vi "Online_Target_3.vi"   [LabVIEW 2021]
uses:
  Model_Updating_Classes/DROPBEAR_Model_Updating/DROPBEAR_Model_Updating.lvclass
types:
  T1 = cluster{"beam_length":dbl, "youngs_modulus":dbl, "torsion_spring":dbl, "beam_height":dbl, "beam_width":dbl, "beam_density":dbl, "number_of_FEA_nodes":i32, "accelerometer_mass":dbl}
  T2 = cluster{"Frequency KF":bool, "Pinned State KF":bool, "FFT Bounding":bool, "Filter Constants Frequency":cluster{"Measurement Variance":dbl, "State Variance":dbl, "Threshold":dbl}, "Filter Constants Position":cluster{"Measurement Variance":dbl, "State Variance":dbl, "Threshold":dbl}, "Moving Window Size":i32, "Time Series buffer":dbl, "Record Time Series Data":bool, "Record Moving Window Data":bool, "Record Online Error Metrics ":bool, "Record Statistics":bool}
  T3 = cluster{"Eigensolver ":enum16{"LabVIEW Cholesky", "LabVIEW General", "LabVIEW Inverse", "LEMP"}, "Models Forcasted":i32, "Max Roller Velocity":dbl, "Max Roller Position Percent":dbl, "Min Roller Position Percent":dbl}
  T4 = cluster{"Dataset":string, "Resample Method":enum16{"Recorded", "Auto Resample", "Custom Resample"}}
  T5 = cluster{"Modeling Parameters input controls":cluster{"beam_length":dbl, "youngs_modulus":dbl, "torsion_spring":dbl, "beam_height":dbl, "beam_width":dbl, "beam_density":dbl, "number_of_FEA_nodes":i32, "accelerometer_mass":dbl}, "Mockbear input controls":cluster{"Dataset":string, "Resample Method":enum16{"Recorded", "Auto Resample", "Custom Resample"}}, "Simulation Parameters input controls":cluster{"Eigensolver ":enum16{"LabVIEW Cholesky", "LabVIEW General", "LabVIEW Inverse", "LEMP"}, "Models Forcasted":i32, "Max Roller Velocity":dbl, "Max Roller Position Percent":dbl, "Min Roller Position Percent":dbl}, "Program Controls":cluster{"Frequency KF":bool, "Pinned State KF":bool, "FFT Bounding":bool, "Filter Constants Frequency":cluster{"Measurement Variance":dbl, "State Variance":dbl, "Threshold":dbl}, "Filter Constants Position":cluster{"Measurement Variance":dbl, "State Variance":dbl, "Threshold":dbl}, "Moving Window Size":i32, "Time Series buffer":dbl, "Record Time Series Data":bool, "Record Moving Window Data":bool, "Record Online Error Metrics ":bool, "Record Statistics":bool}}
  T6 = enum16{"Recorded", "Auto Resample", "Custom Resample"}[]
  T7 = enum16{"LabVIEW Cholesky", "LabVIEW General", "LabVIEW Inverse", "LEMP"}[]
  T8 = cluster{"Modeling Parameters input controls":cluster{"beam_length":dbl, "youngs_modulus":dbl, "torsion_spring":dbl, "beam_height":dbl, "beam_width":dbl, "beam_density":dbl, "number_of_FEA_nodes":i32, "accelerometer_mass":dbl}, "Mockbear input controls":cluster{"Dataset":string, "Resample Method":enum16{"Recorded", "Auto Resample", "Custom Resample"}}, "Simulation Parameters input controls":cluster{"Eigensolver ":enum16{"LabVIEW Cholesky", "LabVIEW General", "LabVIEW Inverse", "LEMP"}, "Models Forcasted":i32, "Max Roller Velocity":dbl, "Max Roller Position Percent":dbl, "Min Roller Position Percent":dbl}, "Program Controls":cluster{"Frequency KF":bool, "Pinned State KF":bool, "FFT Bounding":bool, "Filter Constants Frequency":cluster{"Measurement Variance":dbl, "State Variance":dbl, "Threshold":dbl}, "Filter Constants Position":cluster{"Measurement Variance":dbl, "State Variance":dbl, "Threshold":dbl}, "Moving Window Size":i32, "Time Series buffer":dbl, "Record Time Series Data":bool, "Record Moving Window Data":bool, "Record Online Error Metrics ":bool, "Record Statistics":bool}}[]
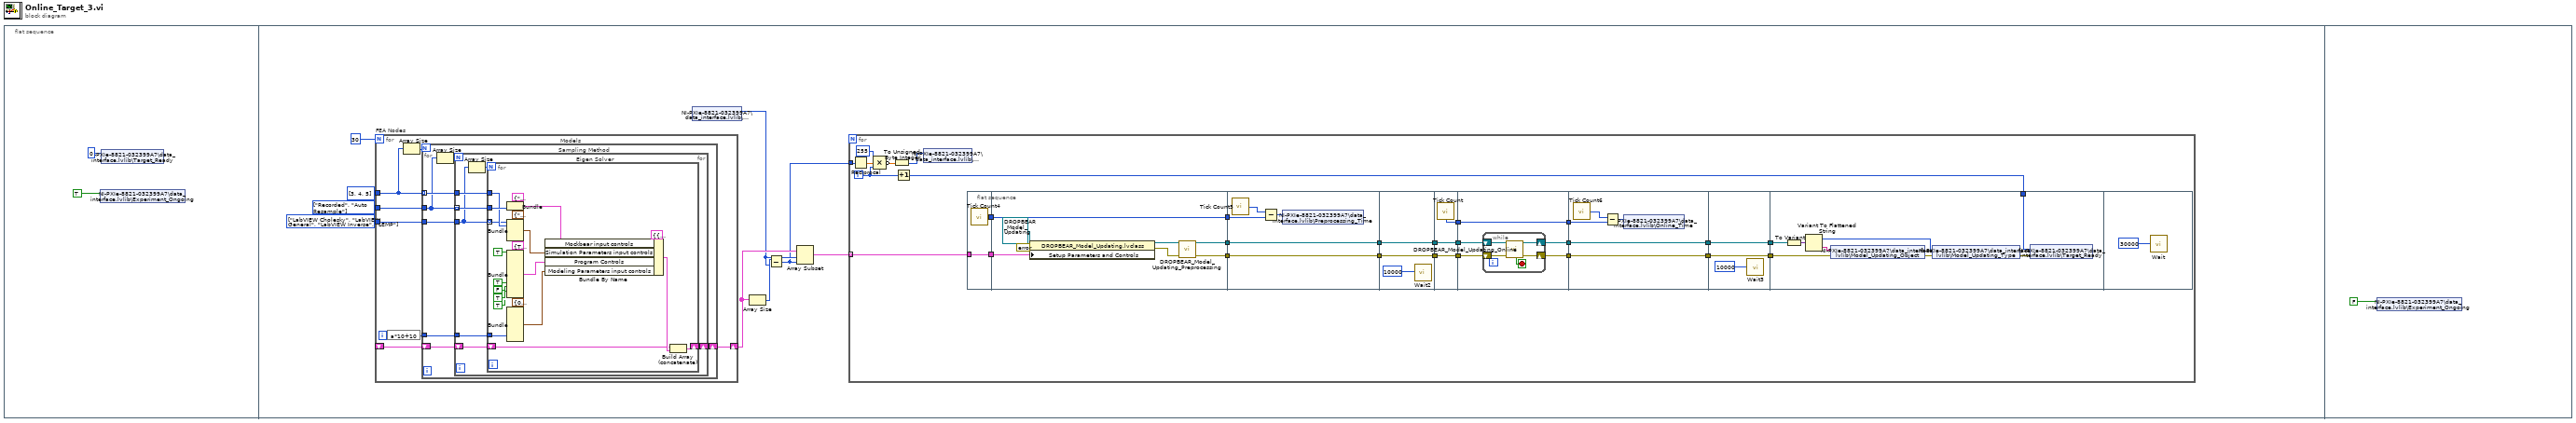
[diagram p0: block diagram]
diagram:
  n1 = flat-sequence {
    frame #0 {
      n2 = shared-variable "NI-PXIe-8821-032399A7\\data_interface.lvlib\\Experiment_Ongoing"(TRUE ("Process_Halt")) -> ()  [unwired: 1 in, 1 out]
      n3 = shared-variable "NI-PXIe-8821-032399A7\\data_interface.lvlib\\Target_Ready"(0) -> ()  [unwired: 1 in, 1 out]
    }
    frame #1 {
      w9 = T6 [enum."Recorded", enum."Auto Resample"] items=["Recorded", "Auto Resample", "Custom Resample"] ("Resample Method")
      w10 = T7 [enum."LabVIEW Cholesky", enum."LabVIEW General", enum."LabVIEW Inverse", enum."LEMP"] items=["LabVIEW Cholesky", "LabVIEW General", "LabVIEW Inverse", "LEMP"] ("Eigensolver")
      n4 = for "FEA Nodes" {
        N: 30 -> [_]
        tunnel: w10 -> [w92]
        tunnel: w9 -> [w91]
        tunnel: i32[] [3, 4, 5] -> [w88]
        shift-right: [w89] -> w7
        shift-left: _ -> [w90]
        i -> [w94]
        n5 = expression code="a*10+10"(w94) -> (w93:i32)
        n6 = Array Size(array=w88) -> (size(s)=w87:i32)
        n7 = for "Models" {
          N: w87 -> [_]
          tunnel: w93 -> [w101]
          tunnel: w92 -> [w100]
          tunnel: w91 -> [w95]
          tunnel: w88 -> [w99] mode=indexing
          shift-right: [w97] -> w89
          shift-left: w90 -> [w98]
          n8 = Array Size(array=w95) -> (size(s)=w96:i32)
          n9 = for "Sampling Method" {
            N: w96 -> [_]
            tunnel: w101 -> [w108]
            tunnel: w100 -> [w102]
            tunnel: w95 -> [w107] mode=indexing
            tunnel: w99 -> [w106]
            shift-right: [w104] -> w97
            shift-left: w98 -> [w105]
            n10 = Array Size(array=w102) -> (size(s)=w103:i32)
            n11 = for "Eigen Solver" {
              N: w103 -> [_]
              tunnel: w108 -> [w115]
              tunnel: w102 -> [w112] mode=indexing
              tunnel: w107 -> [w114]
              tunnel: w106 -> [w113]
              shift-right: [w111] -> w104
              shift-left: w105 -> [w109]
              n12 = Bundle(cluster=T4 {"Dataset"="test7", "Resample Method"=enum."Auto Resample"} ("Mockbear input controls"), "Resample Method"=w114) -> (w123:T4)  [unwired: 1 in]
              n13 = Bundle(cluster=T3 {"Eigensolver "=enum."LEMP", "Models Forcasted"=5, "Max Roller Velocity"=3.32, "Max Roller Position Percent"=0.43, "Min Roller Position Percent"=0.155} ("Simulation Parameters input controls"), "Eigensolver"=w112, "Models Forcasted"=w113) -> (w124:T3)  [unwired: 3 in]
              n14 = Bundle(cluster=T2 {"Frequency KF"=TRUE, "Pinned State KF"=FALSE, "FFT Bounding"=FALSE, "Filter Constants Frequency"={"Measurement Variance"=0.4, "State Variance"=0.01, "Threshold"=1000000000.0}, "Filter Constants Position"={"Measurement Variance"=0.4, "State Variance"=0.9, "Threshold"=1000000000.0}, "Moving Window Size"=10, "Time Series buffer"=10000.0, "Record Time Series Data"=FALSE, "Record Moving Window Data"=FALSE, "Record Online Error Metrics "=TRUE, "Record Statistics"=TRUE} ("Program Controls"), "Frequency KF"=TRUE, "Record Time Series Data"=TRUE, "Record Moving Window Data"=FALSE, "Record Online Error Metrics"=TRUE, "Record Statistics"=TRUE) -> (w129:T2)  [unwired: 6 in]
              n15 = Bundle(cluster=T1 {"beam_length"=0.3525, "youngs_modulus"=209500000000.0, "torsion_spring"=0.0, "beam_height"=0.00635, "beam_width"=0.0508, "beam_density"=7900.0, "number_of_FEA_nodes"=40, "accelerometer_mass"=0.055} ("Modeling Parameters input controls"), "number_of_FEA_nodes"=w115) -> (w121:T1)  [unwired: 7 in]
              n16 = Bundle By Name(cluster=T5 {"Modeling Parameters input controls"={"beam_length"=0.3525, "youngs_modulus"=209500000000.0, "torsion_spring"=0.0, "beam_height"=0.00635, "beam_width"=0.0508, "beam_density"=7900.0, "number_of_FEA_nodes"=40, "accelerometer_mass"=0.055}, "Mockbear input controls"={"Dataset"="test7", "Resample Method"=enum."Auto Resample"}, "Simulation Parameters input controls"={"Eigensolver "=enum."LEMP", "Models Forcasted"=5, "Max Roller Velocity"=3.32, "Max Roller Position Percent"=0.43, "Min Roller Position Percent"=0.155}, "Program Controls"={"Frequency KF"=TRUE, "Pinned State KF"=FALSE, "FFT Bounding"=FALSE, "Filter Constants Frequency"={"Measurement Variance"=0.4, "State Variance"=0.01, "Threshold"=1000000000.0}, "Filter Constants Position"={"Measurement Variance"=0.4, "State Variance"=0.9, "Threshold"=1000000000.0}, "Moving Window Size"=10, "Time Series buffer"=10000.0, "Record Time Series Data"=FALSE, "Record Moving Window Data"=FALSE, "Record Online Error Metrics "=TRUE, "Record Statistics"=TRUE}} ("Setup Parameters and Controls"), "Mockbear input controls"=w123, "Simulation Parameters input controls"=w124, "Program Controls"=w129, "Modeling Parameters input controls"=w121) -> (w110:T5)
              n17 = Build Array (concatenate)(w109, w110) -> (w111:T8)
            }
          }
        }
      }
      n18 = shared-variable "NI-PXIe-8821-032399A7\\data_interface.lvlib\\continue"() -> (w5:i32)  [unwired: 1 in, 1 out]
      n19 = Array Size(array=w7) -> (size(s)=w6:i32)
      n20 = Subtract(x=w6, y=w5) -> (x-y=w3:i32)
      n21 = Array Subset(array=w7, index=w5, length=w3) -> (w4:T8)
      n22 = for {
        tunnel: w4 -> [w25] mode=indexing
        tunnel: w3 -> [w27]
        i -> [w24]
        n23 = Reciprocal(x=w27) -> (1/x=w31:dbl)
        n24 = Compound Arithmetic op=MULTIPLY(255, w31, w24) -> (invert w29:dbl)
        n25 = To Unsigned Byte Integer(number=w29) -> (unsigned 8bit integer=w28:u8)
        n26 = Increment(x=w24) -> (x+1=w23:i32)
        n27 = shared-variable "NI-PXIe-8821-032399A7\\data_interface.lvlib\\Progress"(w28) -> ()  [unwired: 1 in, 1 out]
        n28 = flat-sequence {
          tunnel: [w40] -> w38
          tunnel: [w39] -> w26
          tunnel: w25 -> [w39]
          tunnel: [w44] -> w37
          tunnel: [w43] -> w36
          tunnel: [w42] -> w35
          tunnel: w38 -> [w42]
          tunnel: w26 -> [w41]
          tunnel: w37 -> [w53]
          tunnel: [w53] -> w22
          tunnel: w36 -> [w52]
          tunnel: [w52] -> w21
          tunnel: w35 -> [w50]
          tunnel: w22 -> [w56]
          tunnel: [w56] -> w16
          tunnel: w21 -> [w55]
          tunnel: [w55] -> w14
          tunnel: w16 -> [w59]
          tunnel: [w59] -> w15
          tunnel: w14 -> [w58]
          tunnel: [w58] -> w13
          tunnel: [w57] -> w12
          tunnel: w15 -> [w64]
          tunnel: w13 -> [w63]
          tunnel: [w62] -> w34
          tunnel: [w61] -> w33
          tunnel: [w60] -> w32
          tunnel: w12 -> [w60]
          tunnel: w34 -> [w74]
          tunnel: [w74] -> w20
          tunnel: w33 -> [w73]
          tunnel: [w73] -> w18
          tunnel: w32 -> [w70]
          tunnel: w20 -> [w77]
          tunnel: [w77] -> w19
          tunnel: w18 -> [w76]
          tunnel: [w76] -> w17
          tunnel: w19 -> [w81]
          tunnel: w17 -> [w80]
          tunnel: w23 -> [w78]
          frame #0 {
            n29 = call "Tick Count4"() -> ("Tick Count(uSec)"=w40:u32)
          }
          frame #1 {
            n30 = property class="DROPBEAR_Model_Updating.lvclass"(reference=refnum<class "DROPBEAR_Model_Updating.lvclass"> refnum ("DROPBEAR_Model_Updating.lvclass"), error in=errorcluster {"status"=FALSE, "code"=0, "source"=""} ("error in (no error)"), "Setup Parameters and Controls"=w41) -> (reference out=w48:refnum<class "DROPBEAR_Model_Updating.lvclass">, error out=w45:errorcluster)
            n31 = call-dynamic "DROPBEAR_Model_Updating_Preprocessing.vi"("error in (no error)"=w45, "DROPBEAR_Model_Updating in"=w48) -> ("error out"=w43:errorcluster, "DROPBEAR_Model_Updating out"=w44:refnum<class "DROPBEAR_Model_Updating.lvclass">)  [unwired: 8 in]
          }
          frame #2 {
            n32 = call "Tick Count5"() -> ("Tick Count(uSec)"=w49:u32)
            n33 = Subtract(x=w49, y=w50) -> (x-y=w51:u32)
            n34 = shared-variable "NI-PXIe-8821-032399A7\\data_interface.lvlib\\Preprocessing_Time"(w51) -> ()  [unwired: 1 in, 1 out]
          }
          frame #3 {
            n35 = call "Wait2"("Count(mSec)"=u32 10000) -> ()  [unwired: 1 out]
          }
          frame #4 {
            n36 = call "Tick Count"() -> ("Tick Count(uSec)"=w57:u32)
          }
          frame #5 {
            n37 = while {
              shift-right: [w67] -> w62
              shift-left: w64 -> [w69]
              shift-right: [w66] -> w61
              shift-left: w63 -> [w68]
              stop <- w65 stop-if-true
              n38 = call-dynamic "DROPBEAR_Model_Updating_Online.vi"("error in (no error)"=w68, "DROPBEAR_Model_Updating in"=w69) -> ("error out"=w66:errorcluster, "DROPBEAR_Model_Updating out"=w67:refnum<class "DROPBEAR_Model_Updating.lvclass">, "looping"=w65:bool)  [unwired: 7 in]
            }
          }
          frame #6 {
            n39 = call "Tick Count6"() -> ("Tick Count(uSec)"=w71:u32)
            n40 = Subtract(x=w71, y=w70) -> (x-y=w72:u32)
            n41 = shared-variable "NI-PXIe-8821-032399A7\\data_interface.lvlib\\Online_Time"(w72) -> ()  [unwired: 1 in, 1 out]
          }
          frame #7 {
            n42 = call "Wait3"("Count(mSec)"=u32 10000) -> ()  [unwired: 1 out]
          }
          frame #8 {
            n43 = To Variant(anything=w81) -> (Variant=w82:variant)
            n44 = Variant To Flattened String(Variant=w82) -> (data string=w85:string, 1:w83:i16[])
            n45 = shared-variable "NI-PXIe-8821-032399A7\\data_interface.lvlib\\Model_Updating_Object"(w85, error in=w80) -> (error out=w84:errorcluster)
            n46 = shared-variable "NI-PXIe-8821-032399A7\\data_interface.lvlib\\Model_Updating_Type"(w83, error in=w84) -> (error out=w79:errorcluster)
            n47 = shared-variable "NI-PXIe-8821-032399A7\\data_interface.lvlib\\Target_Ready"(w78, error in=w79) -> ()  [unwired: 1 out]
          }
          frame #9 {
            n48 = call "Wait"("Count(mSec)"=u32 30000) -> ()  [unwired: 1 out]
          }
        }
      }
    }
    frame #2 {
      n49 = shared-variable "NI-PXIe-8821-032399A7\\data_interface.lvlib\\Experiment_Ongoing"(FALSE ("Process_Halt")) -> ()  [unwired: 1 in, 1 out]
    }
  }
